vi "Keithley J-t IIT_v2.vi"(0 "VISA resource name in":refnum<visa-resource-name>, 7 "t=0 timestamp":sgl, 9 "Light?":bool, 11 "Voltage List":dbl[](array[numeric])) -> (4 "VISA resource name out":refnum<visa-resource-name>, 6 "Data Array":dbl[][](array[numeric]), 8 "timestamp":sgl, 15 "Measurement Complete":bool)   [LabVIEW 2011]
doc: "Configures a sweep and takes voltage and current readings at each point."
uses:
  <instrlib>/keithley_24xx/Keithley 24XX/Public/Data/Read (Single Point).vi
  <instrlib>/keithley_24xx/Keithley 24XX/Keithley 24XX.lvlib
panel:
  out "x-y":u32
  in  "Source Mode  (0: Voltage)":u16(ring) items=["Voltage", "Current"]
  # "(c) 2006 National Instruments.  ALL RIGHTS RESERVED."
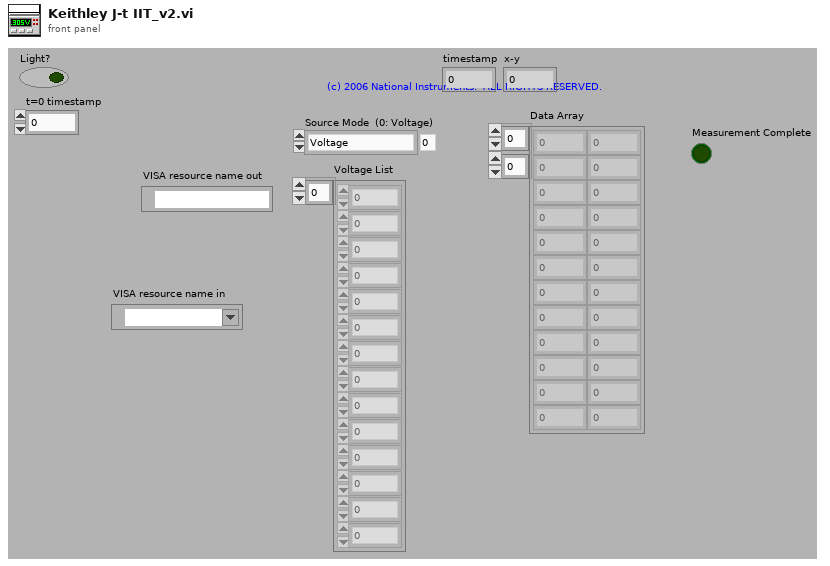
[diagram p1: front panel]
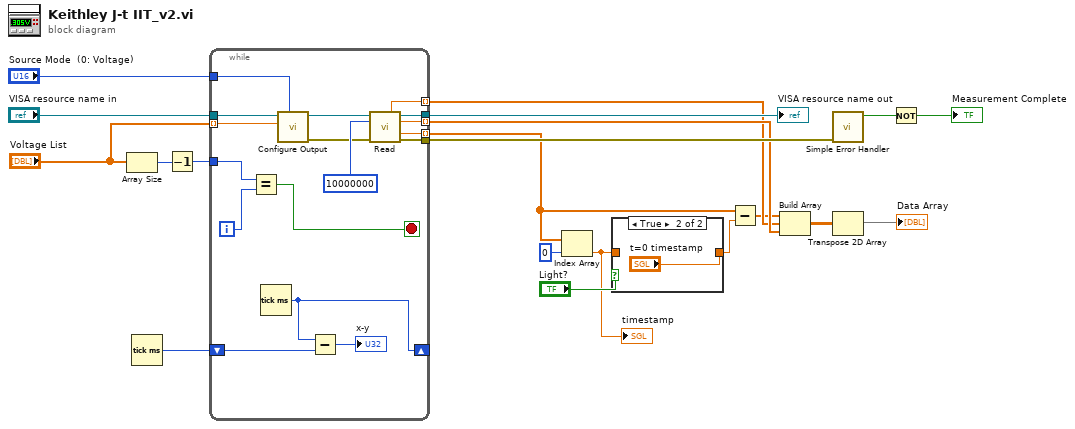
[diagram p0: block diagram]
diagram:
  n1 = Array Size(array="Voltage List") -> (size(s)=w3:i32)
  n2 = Tick Count (ms)() -> (millisecond timer value=w1:u32)
  n3 = Decrement(x=w3) -> (x-1=w2:i32)
  n4 = while {
    tunnel: [w37] -> w20
    tunnel: [w36] -> w19
    tunnel: "VISA resource name in" -> [w32]
    tunnel: "Source Mode  (0: Voltage)" -> [w31]
    tunnel: [w30] -> w14 mode=indexing
    tunnel: "Voltage List" -> [w29] mode=indexing
    tunnel: [w28] -> w13 mode=indexing
    tunnel: [w27] -> w11 mode=indexing
    tunnel: w2 -> [w26]
    shift-right: [w22] -> _
    shift-left: w1 -> [w23]
    i -> [w25]
    stop <- w24 stop-if-true
    n5 = Equal?(x=w26, y=w25) -> (x = y?=w24:bool)
    n6 = Tick Count (ms)() -> (millisecond timer value=w22:u32)
    n7 = call <instrlib>:"Configure Output.vi"("Source Mode  (0: Voltage)"=w31, "Output Level (0)"=w29, "VISA resource name"=w32) -> ("error out"=w33:errorcluster, "VISA resource name out"=w34:refnum<visa-resource-name>)  [unwired: 7 in]
    n8 = Subtract(x=w22, y=w23) -> (x-y=→"x-y":u32)
    n9 = call-poly <instrlib>:"Read.vi"("VISA resource name"=w34, "Timeout (10000 ms)"=10000000, "error in (no error)"=w33) -> ("Voltage"=w28:sgl, "VISA resource name out"=w36:refnum<visa-resource-name>, "Current"=w30:sgl, "Timestamp"=w27:sgl, "error out"=w37:errorcluster)  [unwired: 6 in, 2 out]
  }
  "VISA resource name out" <- w19
  n10 = Index Array(array=w11, index=0) -> (element=w7:sgl)
  "timestamp" <- w7
  n11 = case shown="True" "Light?" {
    tunnel: [w38 "t=0 timestamp"] -> w8
    tunnel: w7 -> [w38 _]
    frame False {
    }
    frame True {
    }
  }
  n12 = Subtract(x=w11, y=w8) -> (x-y=w12:sgl[])
  n13 = Build Array(w12, w13, w14) -> (w6:sgl[][])
  n14 = call <vilib>:"Simple Error Handler.vi"("error in (no error)"=w20) -> ("error?"=w18:bool)  [unwired: 4 in, 4 out]
  n15 = Transpose 2D Array(2D array=w6) -> (transposed array=→"Data Array":sgl[][])
  n16 = Not(x=w18) -> (.not. x?=→"Measurement Complete":bool)
